vi "No-op Encoder.vi"(11 "Value":string) -> (0 "error out":errorcluster, 3 "Canonicalized Protocol":string)   [LabVIEW 2020, in "Stream.lvlib" / "URLPattern.lvclass"]
uses:
  URLPattern.lvclass
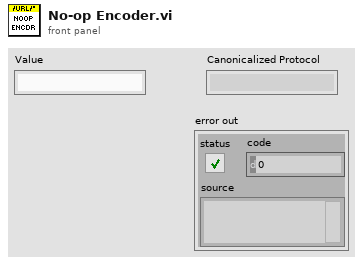
[diagram p1: front panel]
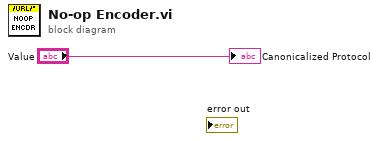
[diagram p0: block diagram]
diagram:
  "Canonicalized Protocol" <- "Value"
